vi "Template.vi"() -> ()   [LabVIEW 2025]
uses:
  _Template/_Template/_Template.lvclass
  _Shared/_Shared.lvlib
  _Shared/Panel/Panel.lvlib
  _Shared/Tree/Tree.lvlib
panel:
  out "Target":string
  in  "Tree":string(tree)
  in  "OK":bool
  # "Disclaimer: Please consider committing changes before AND after this action"
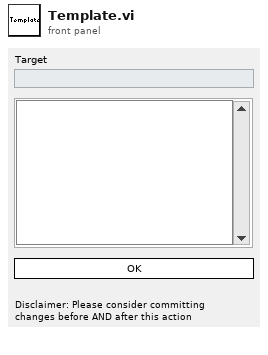
[diagram p1: front panel]
types:
  T1 = typedef "_Shared.lvlib/Type Name Library File Path.ctl" = map{T2, T3}
  T2 = typedef "_Shared.lvlib/Type.ctl" = enum16{"Actor", "Msg"}
  T3 = typedef "_Shared.lvlib/Name Library File Path.ctl" = map{string, path}
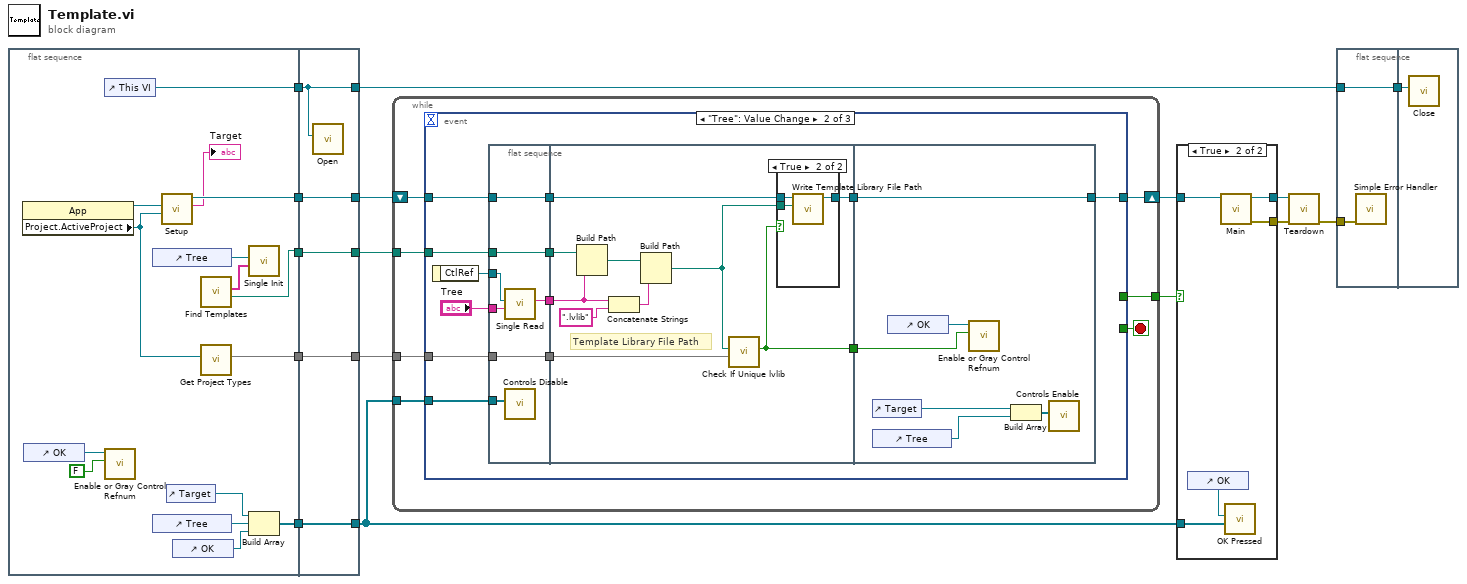
[diagram p0: block diagram]
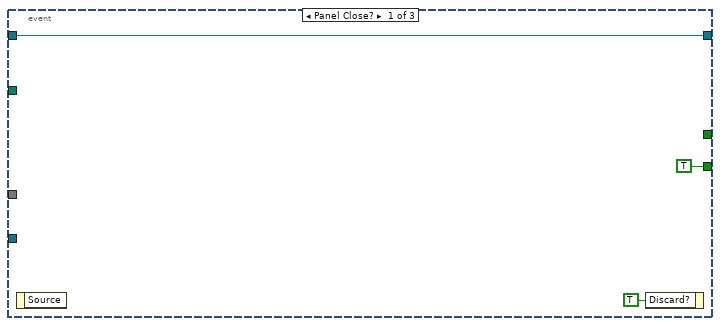
[diagram p2: hidden frame]
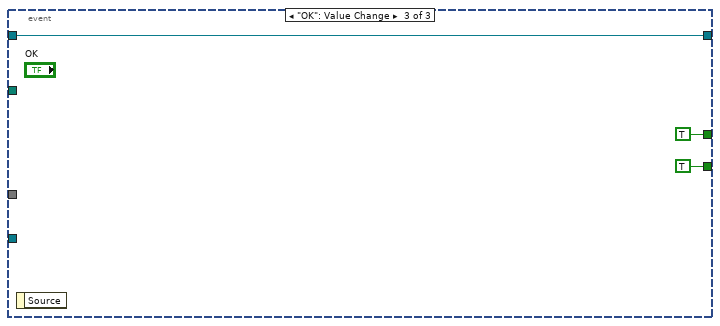
[diagram p4: hidden frame]
diagram:
  n1 = flat-sequence {
    tunnel: [w31] -> w14
    tunnel: [w30] -> w13
    tunnel: [w28] -> w12
    tunnel: [w25] -> w8
    tunnel: [w20] -> w4
    tunnel: [w36] -> w10
    tunnel: w14 -> [w36]
    tunnel: w13 -> [w35]
    tunnel: [w35] -> w6
    tunnel: [w34] -> w11
    tunnel: w12 -> [w34]
    tunnel: [w33] -> w9
    tunnel: w8 -> [w33]
    tunnel: [w32] -> w5
    tunnel: w4 -> [w32]
    frame #0 {
      n2 = property class="App"() -> (reference out=w27:refnum<vi>, "Project.ActiveProject"=w26:refnum<vi>)  [unwired: 2 in, 1 out]
      n3 = control-ref of="OK"() -> (w23:refnum<vi>)
      n4 = control-ref of="This VI"() -> (w30:refnum<vi>)
      n5 = call <vilib>:"Enable or Gray Control Refnum.vi"("enable?"=FALSE, "Control in"=w23) -> ()  [unwired: 8 in, 2 out]
      n6 = control-ref of="Tree"() -> (w21:refnum<vi>)
      n7 = control-ref of="Tree"() -> (w24:refnum<vi>)
      n8 = call "Setup.vi"("Active Project"=w26, "NI.LV.Dialog Instance"=w27) -> ("Target"=→"Target":string, "_Template out"=w25:refnum<class "_Template.lvclass">)  [unwired: 8 in]
      n9 = control-ref of="Target"() -> (w17:refnum<vi>)
      n10 = control-ref of="OK"() -> (w29:refnum<vi>)
      n11 = call "Find Templates.vi"() -> ("Template Path"=w20:path, "List Folders"=w19:string[])  [unwired: 10 in]
      n12 = call "Get Project Types.vi"("Project:Active Project"=w26) -> ("Type Name Library File Path"=w31:T1)  [unwired: 10 in]
      n13 = call "Single Init.vi"("Left Cell Strings"=w19, "Tree Ref"=w21) -> ()  [unwired: 10 in]
      n14 = Build Array(w17, w24, w29) -> (w28:refnum<vi>[])
    }
    frame #1 {
      n15 = call "Open.vi"("VI"=w35) -> ()  [unwired: 11 in]
    }
  }
  n16 = while {
    tunnel: [w43] -> w16
    shift-right: [w40] -> w15
    shift-left: w9 -> [w41]
    tunnel: w5 -> [w39]
    tunnel: w10 -> [w38]
    tunnel: w11 -> [w37]
    stop <- w42 stop-if-true
    n17 = event shown="[1] \"Tree\": Value Change" {
      selector: _ -> [_ _ _]
      dyn-events: _ -> [_ _ _]
      timeout: _ -> [_ _ _]
      tunnel: [_ _ TRUE] -> w43
      tunnel: [TRUE ("Discard?") _ TRUE ("Discard?")] -> w42
      tunnel: w41 -> [w44 w53 w87]
      tunnel: [w44 w51 w87] -> w40
      tunnel: w39 -> [_ w55 _]
      tunnel: w38 -> [_ w57 _]
      tunnel: w37 -> [_ w59 _]
      event Panel Close? {
        n18 = event-data() -> ()  [unwired: 1 in, 1 out]
        n19 = event-data("Discard?"=TRUE) -> ()  [unwired: 1 in, 1 out]
      }
      event "Tree": Value Change {
        n20 = event-data() -> ("CtlRef"=w47:refnum<vi>)  [unwired: 1 in]
        n21 = flat-sequence {
          tunnel: w59 -> [w66]
          tunnel: [w65] -> w58
          tunnel: w57 -> [w65]
          tunnel: [w63] -> w56
          tunnel: w55 -> [w63]
          tunnel: [w64] -> w54
          tunnel: w53 -> [w64]
          tunnel: [w60] -> w52
          tunnel: "Tree" -> [w61]
          tunnel: w47 -> [w62]
          tunnel: w58 -> [w68]
          tunnel: w56 -> [w73]
          tunnel: w54 -> [w71]
          tunnel: w52 -> [w72]
          tunnel: [w70] -> w50
          tunnel: [w67] -> w49
          tunnel: [w86] -> w51
          tunnel: w50 -> [w86]
          tunnel: w49 -> [w84]
          frame #0 {
            n22 = call "Single Read.vi"("Tree"=w61, "Tree Ref"=w62) -> ("Name"=w60:string)  [unwired: 9 in]
            n23 = call "Controls Disable.vi"("Controls in"=w66) -> ()  [unwired: 11 in]
          }
          frame #1 {
            # "Template Library File Path"
            n24 = Build Path(base path=w73, name or relative path=w72) -> (appended path=w75:path)
            n25 = Concatenate Strings(w72, ".lvlib" ("string")) -> (w76:string)
            n26 = Build Path(base path=w75, name or relative path=w76) -> (appended path=w69:path)
            n27 = call "Check If Unique lvlib.vi"("Type Name Library File Path"=w68, "Library File Path"=w69) -> ("Unique?"=w67:bool)  [unwired: 9 in]
            n28 = case shown="True" w67 {
              tunnel: w71 -> [w77 w80]
              tunnel: [w77 w79] -> w70
              tunnel: w69 -> [_ w78]
              frame False {
              }
              frame True {
                n29 = call "Write Template Library File Path.vi"("Template Library File Path"=w78, "_Template in"=w80) -> ("_Template out"=w79:refnum<class "_Template.lvclass">)  [unwired: 9 in]
              }
            }
          }
          frame #2 {
            n30 = control-ref of="Target"() -> (w83:refnum<vi>)
            n31 = control-ref of="Tree"() -> (w82:refnum<vi>)
            n32 = control-ref of="OK"() -> (w85:refnum<vi>)
            n33 = call <vilib>:"Enable or Gray Control Refnum.vi"("enable?"=w84, "Control in"=w85) -> ()  [unwired: 8 in, 2 out]
            n34 = Build Array(w83, w82) -> (w81:refnum<vi>[])
            n35 = call "Controls Enable.vi"("Controls in"=w81) -> ()  [unwired: 11 in]
          }
        }
      }
      event "OK": Value Change {
        n36 = event-data() -> ()  [unwired: 1 in, 1 out]
      }
    }
  }
  n37 = case shown="True" w16 {
    tunnel: w15 -> [w90 w92]
    tunnel: [_ w95] -> w3
    tunnel: w11 -> [_ w93]
    tunnel: [w90 w91] -> w1
    frame False {
    }
    frame True {
      n38 = control-ref of="OK"() -> (w94:refnum<vi>)
      n39 = call "Main.vi"("_Template in"=w92) -> ("error out"=w95:errorcluster, "_Template out"=w91:refnum<class "_Template.lvclass">)  [unwired: 9 in]
      n40 = call "OK Pressed.vi"("Controls in"=w93, "OK Ref"=w94) -> ()  [unwired: 10 in]
    }
  }
  n41 = call "Teardown.vi"("error in (no error)"=w3, "_Template in"=w1) -> ("error out"=w2:errorcluster)  [unwired: 9 in]
  n42 = flat-sequence {
    tunnel: w2 -> [w97]
    tunnel: w6 -> [w96]
    tunnel: [w96] -> w7
    tunnel: w7 -> [w98]
    frame #0 {
      n43 = call <vilib>:"Simple Error Handler.vi"("error in (no error)"=w97) -> ()  [unwired: 4 in, 5 out]
    }
    frame #1 {
      n44 = call "Close.vi"("VI"=w98) -> ()  [unwired: 11 in]
    }
  }
